vi "ExpEval_ComparePrecedence.vi"(10 "Operator 2":string, 11 "Operator 1":string) -> (2 "error":bool, 3 "higher precedence":bool)   [LabVIEW 2017, in "ExpressionEvaluator.lvlib"]
uses:
  <vilib>/addons/InsightCM/Utilities/ExpressionEvaluator/ExpressionEvaluator.lvlib
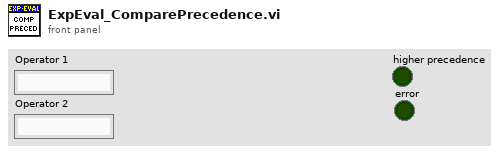
[diagram p1: front panel]
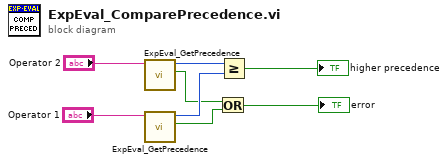
[diagram p0: block diagram]
diagram:
  n1 = call <vilib>:"ExpEval_GetPrecedence.vi"("Operator"="Operator 2") -> ("Not found"=w4:bool, "Precedence"=w6:i32)  [unwired: 9 in]
  n2 = call <vilib>:"ExpEval_GetPrecedence.vi"("Operator"="Operator 1") -> ("Not found"=w3:bool, "Precedence"=w5:i32)  [unwired: 9 in]
  n3 = Or(x=w4, y=w3) -> (x .or. y?=→"error":bool)
  n4 = Greater Or Equal?(x=w6, y=w5) -> (x >= y?=→"higher precedence":bool)
